vi "Delay if no error.vi"(1 "error in (no error)":errorcluster, 4 "milliseconds to wait (1 ms)":u32=1, 8 "Enable? (T)":bool=TRUE) -> (15 "error out":errorcluster)   [LabVIEW 2011]
doc: "Insert a delay with error pass-through to provide data-flow control. Doesn't delay if there is an error in.\n\n\nVersion 1.0 - 10/21/2009\n\nPhaeron, Inc.\nwww.phaeron.com\ninfo@phaeron.com"
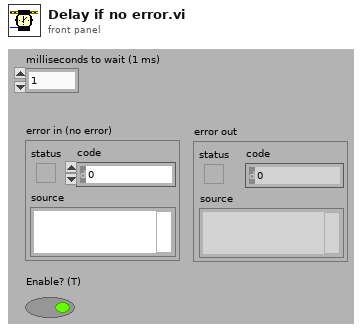
[diagram p1: front panel]
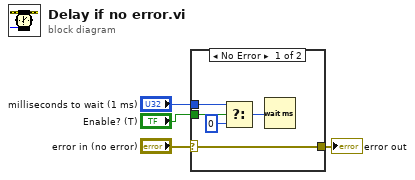
[diagram p0: block diagram]
diagram:
  n1 = case shown="No Error" "error in (no error)" {
    selector: "error in (no error)" -> [w9 w10]
    tunnel: "milliseconds to wait (1 ms)" -> [w7 _]
    tunnel: [w9 w10] -> w2
    tunnel: "Enable? (T)" -> [w8 _]
    frame No Error {
      n2 = Select(t=w7, s=w8, f=u32 0) -> (s? t:f=w6:u32)
      n3 = Wait (ms)(milliseconds to wait=w6) -> ()  [unwired: 1 out]
    }
    frame Error {
    }
  }
  "error out" <- w2
